vi "Match Pattern.vi"(6 "trim back if found":i32, 9 "regular expression":string, 10 "Offset in":i32, 11 "String in":string) -> (1 "substring":string, 2 "Offset of match":i32, 3 "Found":bool)   [LabVIEW 2017, in "JSONtext.lvlib"]
uses:
  JSONtext.lvlib
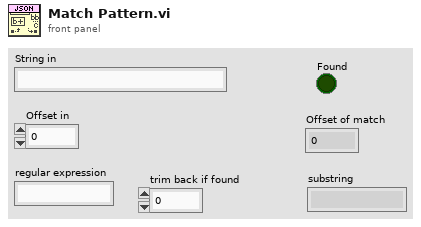
[diagram p1: front panel]
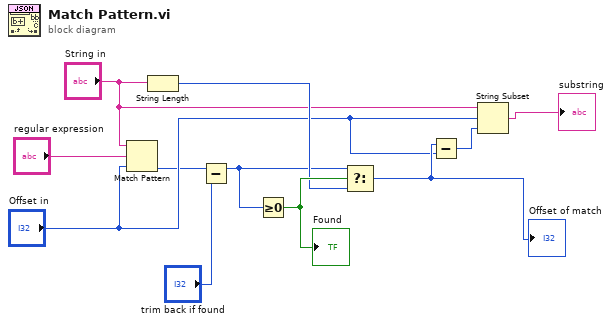
[diagram p0: block diagram]
diagram:
  n1 = Match Pattern(string="String in", regular expression="regular expression", offset (0)="Offset in") -> (offset past match=w4:i32)  [unwired: 3 out]
  n2 = String Length(string="String in") -> (length=w9:i32)
  n3 = Subtract(x=w4, y="trim back if found") -> (x-y=w2:i32)
  n4 = Greater Or Equal To 0?(x=w2) -> (x >= 0?=w11:bool)
  "Found" <- w11
  n5 = Select(t=w2, s=w11, f=w9) -> (s? t:f=w7:i32)
  "Offset of match" <- w7
  n6 = Subtract(x=w7, y="Offset in") -> (x-y=w3:i32)
  n7 = String Subset(string="String in", offset (0)="Offset in", length (rest)=w3) -> (substring=→"substring":string)
